vi "email conversion report.vi"(8 "error in (no error)":errorcluster, 9 "correct number of subfolders":i32, 10 "Array":dbl[][](array[numeric]), 11 "TomoConversion in":refnum<class "TomoConversion.lvclass">) -> (0 "error out":errorcluster, 3 "TomoConversion out":refnum<class "TomoConversion.lvclass">)   [LabVIEW 2012, in "TomoConversion.lvclass"]
uses:
  TomoConversion.lvclass
  TomoConversion.lvclass/TomoConversion.ctl
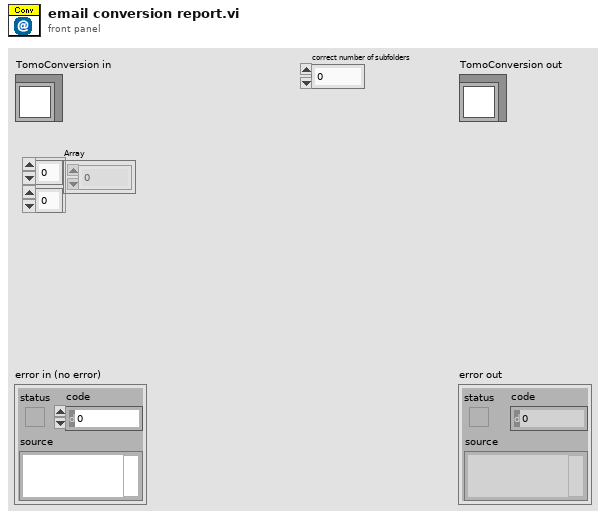
[diagram p1: front panel]
types:
  T1 = typedef "TomoConversion.lvclass/notice type.ctl" = enum16{"Grotto", "folder issue"}
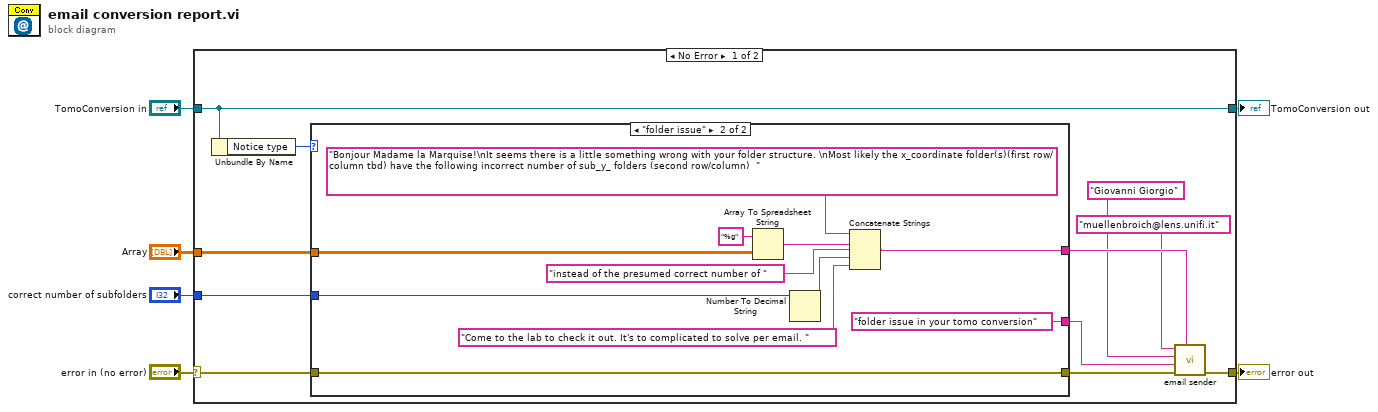
[diagram p0: block diagram]
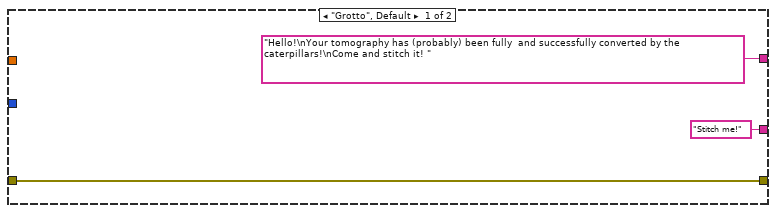
[diagram p2: hidden frame]
diagram:
  n1 = case shown="No Error" "error in (no error)" {
    selector: "error in (no error)" -> [w12 w33]
    tunnel: [w17 w33] -> w5
    tunnel: [w16 w32] -> w3
    tunnel: "TomoConversion in" -> [w16 w32]
    tunnel: "Array" -> [w8 _]
    tunnel: "correct number of subfolders" -> [w7 _]
    frame No Error {
      n2 = Unbundle By Name(w16) -> ("Notice type"=w15:T1)
      n3 = case shown="\"folder issue\"" w15 {
        tunnel: ["Hello!\nYour tomography has (probably) been fully  and successfully converted by the caterpillars!\nCome and stitch it! " w22] -> w14
        tunnel: ["Stitch me!" "folder issue in your tomo conversion"] -> w13
        tunnel: w12 -> [w18 w31]
        tunnel: [w18 w31] -> w11
        tunnel: w8 -> [_ w29]
        tunnel: w7 -> [_ w26]
        frame "Grotto", Default {
        }
        frame "folder issue" {
          n4 = Array To Spreadsheet String(array=w29, 3:"%g" ("format string")) -> (spreadsheet string=w27:string)  [unwired: 1 in]
          n5 = Number To Decimal String(number=w26) -> (decimal integer string=w24:string)  [unwired: 1 in]
          n6 = Concatenate Strings("Bonjour Madame la Marquise!\nIt seems there is a little something wrong with your folder structure. \nMost likely the x_coordinate folder(s)(first row/column tbd) have the following incorrect number of sub_y_ folders (second row/column)  ", w27, "instead of the presumed correct number of " ("string"), w24, "Come to the lab to check it out. It's to complicated to solve per email. " ("string")) -> (w22:string)
        }
      }
      n7 = call "email sender.vi"("Body"=w14, "error in (no error)"=w11, "Subject"=w13, "Recipient's Name"="Giovanni Giorgio", "Recipient's Email Address Address"="muellenbroich@lens.unifi.it") -> ("error out"=w17:errorcluster)  [unwired: 6 in]
    }
    frame Error {
    }
  }
  "error out" <- w5
  "TomoConversion out" <- w3
